vi "Read Result File Path.vi"(8 "error in (no error)":errorcluster, 11 "Charact Result Accessor in":refnum<class "Charact Result Accessor.lvclass">) -> (0 "error out":errorcluster, 2 "Result File Path":path, 3 "Charact Result Accessor out":refnum<class "Charact Result Accessor.lvclass">)   [LabVIEW 2023, in "RFFixtureCharact.RFPM.lvlib" / "Charact Result Accessor.lvclass"]
uses:
  Charact Result Accessor.lvclass
  Charact Result Accessor.lvclass/Charact Result Accessor.ctl
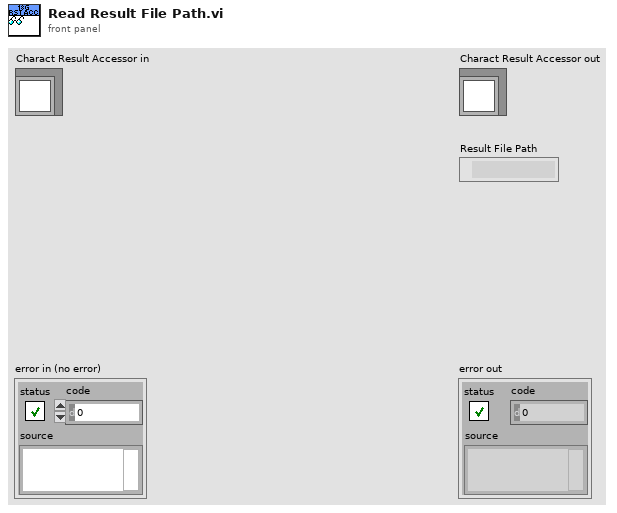
[diagram p1: front panel]
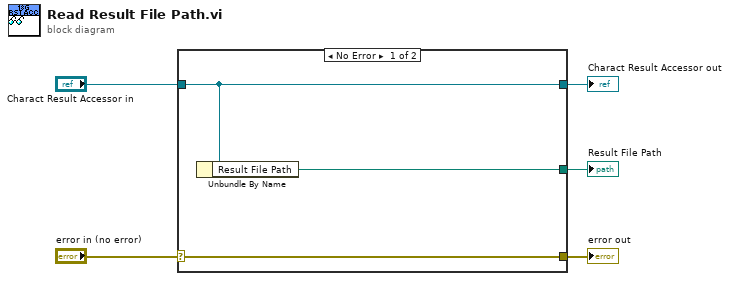
[diagram p0: block diagram]
diagram:
  n1 = case shown="No Error" "error in (no error)" {
    selector: "error in (no error)" -> [w8 w9]
    tunnel: [w8 w9] -> w4
    tunnel: [w7 w10] -> w2
    tunnel: "Charact Result Accessor in" -> [w7 w10]
    tunnel: [w6 _] -> w1
    frame No Error {
      n2 = Unbundle By Name(w7) -> ("Result File Path"=w6:path)
    }
    frame Error {
    }
  }
  "error out" <- w4
  "Charact Result Accessor out" <- w2
  "Result File Path" <- w1
